vi "TcpCommunicationServerModule.vi"(7 "States":T1=enum."Status Check", 8 "エラー入力（エラーなし）":errorcluster, 10 "ポート":u16=8501) -> (0 "エラー出力":errorcluster, 1 "接続数":i32, 3 "Data出力":T2, 5 "Stoped":bool)   [LabVIEW 2017]
uses:
  TcpCommunicationServerData.ctl
  TcpCommunicationServerCMD.ctl
panel:
  out "ReadData":string
  # "サーバ用TCP通信モジュール"
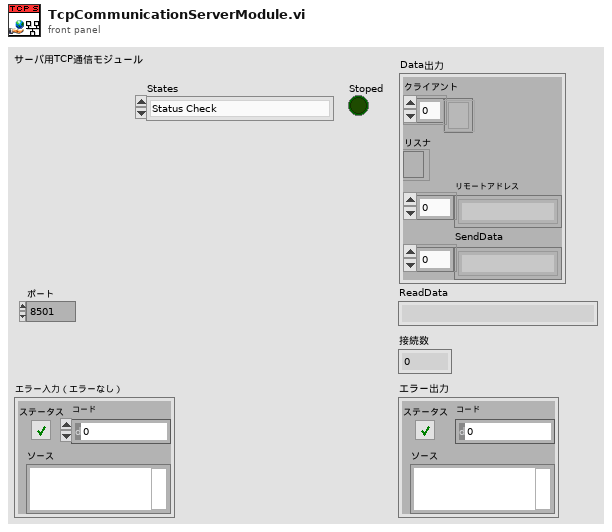
[diagram p1: front panel]
types:
  T1 = typedef "TcpCommunicationServerCMD.ctl" = enum16{"Initialize", "Status Check", "Send Data", "Read Data", "Stop", "GetData"}
  T2 = typedef "TcpCommunicationServerData.ctl" = cluster{"クライアント":refnum<k5>[], "リスナ":refnum<k5>, "リモートアドレス":string[], "SendData":string[]}
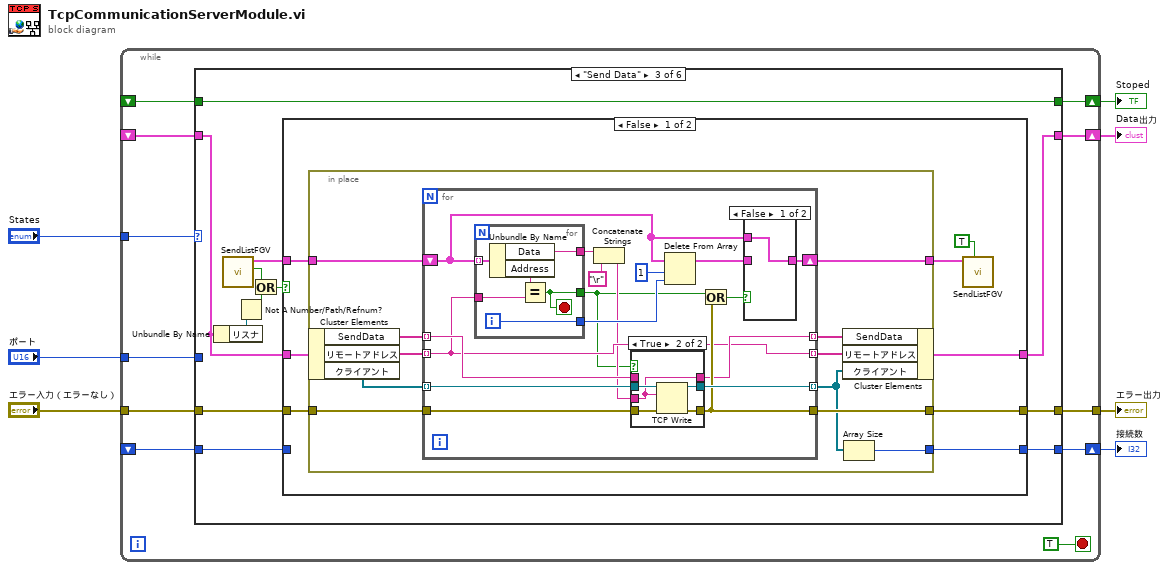
[diagram p0: block diagram]
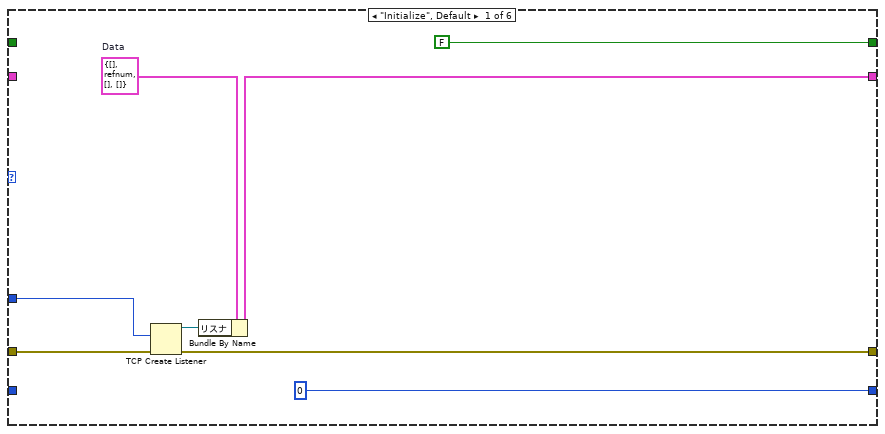
[diagram p2: hidden frame]
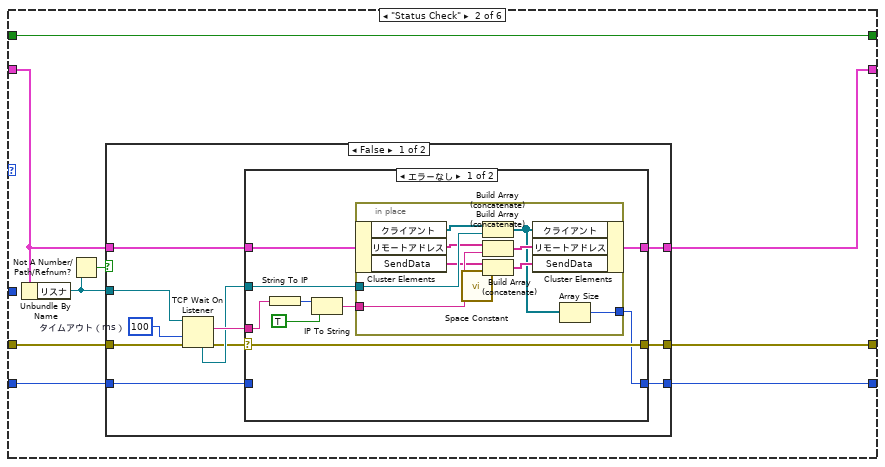
[diagram p3: hidden frame]
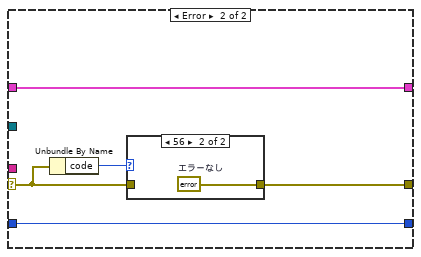
[diagram p4: hidden frame]
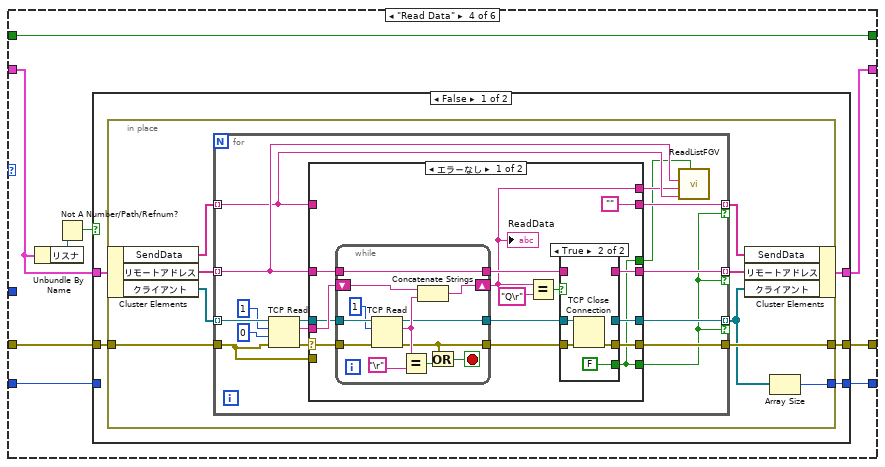
[diagram p10: hidden frame]
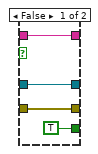
[diagram p11: hidden frame]
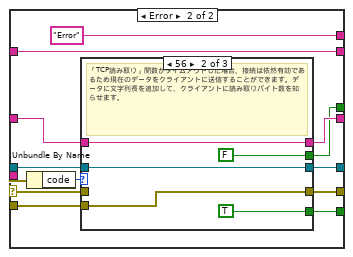
[diagram p12: hidden frame]
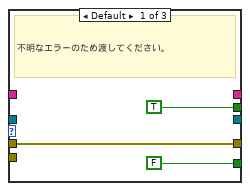
[diagram p13: hidden frame]
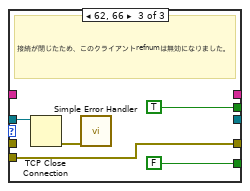
[diagram p14: hidden frame]
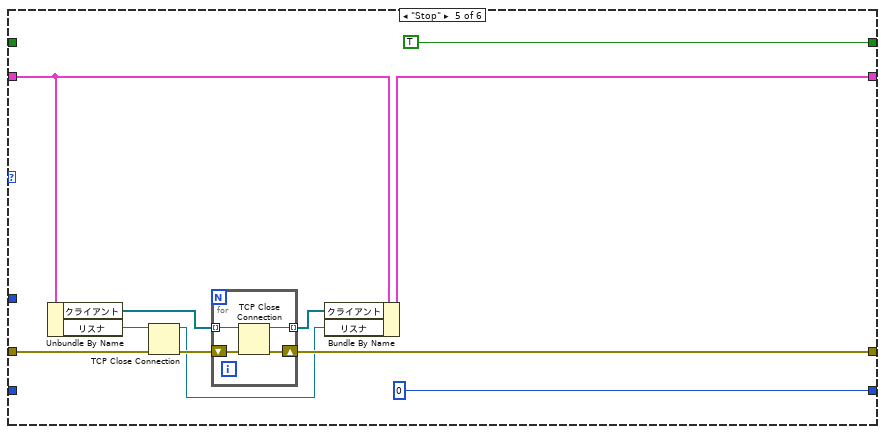
[diagram p16: hidden frame]
diagram:
  n1 = while {
    tunnel: "ポート" -> [w18]
    shift-right: [w17] -> w6
    shift-left: _ -> [w16]
    tunnel: "States" -> [w12]
    shift-right: [w10] -> w1
    shift-left: _ -> [w9]
    shift-right: [w11] -> w2
    shift-left: _ -> [w8]
    tunnel: "エラー入力（エラーなし）" -> [w14]
    tunnel: [w15] -> w5
    stop <- TRUE stop-if-true
    n2 = case shown="\"Send Data\"" w12 {
      tunnel: w18 -> [w26 _ _ _ _ _]
      tunnel: [w24 w34 w83 w148 w247 w262] -> w17
      tunnel: w16 -> [_ w32 w79 w145 w251 w262]
      tunnel: [w23 w33 w84 w150 w250 w261] -> w15
      tunnel: w14 -> [w22 w35 w85 w151 w252 w261]
      tunnel: [0 w31 w82 w149 0 w260] -> w11
      tunnel: [FALSE w30 w81 w147 TRUE w263] -> w10
      tunnel: w9 -> [_ w30 w81 w147 _ w263]
      tunnel: w8 -> [_ w29 w80 w143 _ w260]
      frame "Initialize", Default {
        w21 = T2 {"クライアント"=[], "リスナ"=refnum, "リモートアドレス"=[], "SendData"=[]}  # Data
        n3 = TCP Create Listener(8:w22, 10:w26) -> (0:w23:errorcluster, 3:w25:refnum<k5>)  [unwired: 4 out]
        n4 = Bundle By Name(cluster=w21, "リスナ"=w25) -> (w24:T2)
      }
      frame "Status Check" {
        n5 = Unbundle By Name(w32) -> ("リスナ"=w27:refnum<k5>)
        n6 = Not A Number/Path/Refnum?(number/path/refnum=w27) -> (NaN/Path/Refnum?=w28:bool)
        n7 = case shown="FALSE" w28 {
          tunnel: w27 -> [w45 _]
          tunnel: w35 -> [w41 w74]
          tunnel: [w40 w75] -> w34
          tunnel: [w39 w74] -> w33
          tunnel: w32 -> [w38 w75]
          tunnel: [w37 w73] -> w31
          tunnel: w29 -> [w36 w73]
          frame False {
            w42 = 100  # タイムアウト（ms）
            n8 = TCP Wait On Listener(8:w41, 9:w42, 11:w45) -> (0:w43:errorcluster, 2:w46:string, 4:w44:refnum<k5>)  [unwired: 3 out]
            n9 = case shown="エラーなし" w43 {
              selector: w43 -> [w53 w70]
              tunnel: w44 -> [w54 _]
              tunnel: w38 -> [w55 w67]
              tunnel: [w52 w67] -> w40
              tunnel: [w53 w68] -> w39
              tunnel: w46 -> [w49 _]
              tunnel: [w47 w66] -> w37
              tunnel: w36 -> [_ w66]
              frame No Error {
                # "新規クライアント接続をステートデータに追加して、「データを送信」ステートに進みます。"
                n10 = String To IP(1:w49) -> (0:w51:u32)
                n11 = IP To String(1:TRUE ("ドット表記法?（F）"), 2:w51) -> (0:w48:string)
                n12 = in-place {
                  in-place-border: w54 -> [w64]
                  in-place-border: w48 -> [w61]
                  in-place-border: [w56] -> w47
                  n13 = in-place-cluster #1(w55) -> ("クライアント"=w65:refnum<k5>[], "リモートアドレス"=w63:string[], "SendData"=w59:string[])
                  n14 = call <vilib>:"Space Constant.vi"() -> ("String"=w58:string)
                  n15 = Build Array (concatenate)(w65, w64) -> (w57:refnum<k5>[])
                  n16 = Build Array (concatenate)(w63, w61) -> (w62:string[])
                  n17 = Build Array (concatenate)(w59, w58) -> (w60:string[])
                  n18 = in-place-cluster #1("クライアント"=w57, "リモートアドレス"=w62, "SendData"=w60) -> (w52:T2)
                  n19 = Array Size(array=w57) -> (size(s)=w56:i32)
                }
              }
              frame Error {
                # "タイムアウトエラーを無視します。クライアントが存在する場合は、「データを送信」ステートに進みます。"
                n20 = Unbundle By Name(w70) -> ("code"=w69:i32)
                n21 = case shown="56" w69 {
                  tunnel: w70 -> [w71 _]
                  tunnel: [w71 w72] -> w68
                  frame Default {
                  }
                  frame 56 {
                    w72 = errorcluster {"status"=FALSE, "code"=0, "source"=""}  # エラーなし
                  }
                }
              }
            }
          }
          frame True {
          }
        }
      }
      frame "Send Data" {
        n22 = Unbundle By Name(w79) -> ("リスナ"=w78:refnum<k5>)
        n23 = call "SendListFGV.vi"() -> ("空?"=w86:bool, "Send List Out"=w87:cluster{"Address":string, "Data":string}[])  [unwired: 9 in, 1 out]
        n24 = Not A Number/Path/Refnum?(number/path/refnum=w78) -> (NaN/Path/Refnum?=w76:bool)
        n25 = Or(x=w86, y=w76) -> (x .or. y?=w77:bool)
        n26 = case shown="FALSE" w77 {
          tunnel: w85 -> [w95 w142]
          tunnel: [w94 w142] -> w84
          tunnel: w79 -> [w93 w141]
          tunnel: [w92 w141] -> w83
          tunnel: w87 -> [w90 _]
          tunnel: [w91 w140] -> w82
          tunnel: w80 -> [_ w140]
          frame False {
            n27 = in-place {
              in-place-border: w95 -> [w106]
              in-place-border: [w105] -> w94
              in-place-border: [w98] -> w91
              in-place-border: w90 -> [w97]
              in-place-border: [w96] -> w88
              n28 = in-place-cluster #2(w93) -> ("SendData"=w99:string[], "リモートアドレス"=w102:string[], "クライアント"=w104:refnum<k5>[])
              n29 = for {
                tunnel: w104 -> [w123] mode=indexing
                tunnel: [w122] -> w103 mode=indexing
                tunnel: w102 -> [w117] mode=indexing
                tunnel: [w117] -> w101 mode=indexing
                tunnel: [w119] -> w100 mode=indexing
                tunnel: w99 -> [w118] mode=indexing
                tunnel: w106 -> [w121]
                tunnel: [w120] -> w105
                shift-right: [w109] -> w96
                shift-left: w97 -> [w110]
                n30 = for {
                  tunnel: w110 -> [w128] mode=indexing
                  tunnel: w117 -> [w131]
                  tunnel: [w129] -> w116
                  tunnel: [w127] -> w107
                  tunnel: [w126] -> w114
                  i -> [w126]
                  stop <- w127 stop-if-true
                  n31 = Unbundle By Name(w128) -> ("Data"=w129:string, "Address"=w130:string)
                  n32 = Equal?(x=w130, y=w131) -> (x = y?=w127:bool)
                }
                n33 = Concatenate Strings(w116, "\r") -> (w112:string)
                n34 = case shown="TRUE" w107 {
                  tunnel: w123 -> [w134 w139]
                  tunnel: [w134 w138] -> w122
                  tunnel: [w133 w137] -> w120
                  tunnel: w121 -> [w133 w136]
                  tunnel: w112 -> [_ w135]
                  tunnel: w118 -> [w132 _]
                  tunnel: [w132 w135] -> w119
                  frame False {
                  }
                  frame True {
                    n35 = TCP Write(connection ID=w139, data in=w135, error in (no error)=w136) -> (connection ID out=w138:refnum<k5>, error out=w137:errorcluster)  [unwired: 2 out]
                  }
                }
                n36 = Delete From Array(array=w110, length=1 ("長さ"), index=w114) -> (array with subset deleted=w111:cluster{"Address":string, "Data":string}[])  [unwired: 1 out]
                n37 = Or(x=w107, y=w120) -> (x .or. y?=w108:bool)
                n38 = case shown="FALSE" w108 {
                  tunnel: w110 -> [w124 _]
                  tunnel: [w124 w125] -> w109
                  tunnel: w111 -> [_ w125]
                  frame False {
                  }
                  frame True {
                  }
                }
              }
              n39 = in-place-cluster #2("SendData"=w100, "リモートアドレス"=w101, "クライアント"=w103) -> (w92:T2)
              n40 = Array Size(array=w103) -> (size(s)=w98:i32)
            }
            n41 = call "SendListFGV.vi"("Set"=TRUE, "Send List"=w88) -> ()  [unwired: 7 in, 3 out]
          }
          frame True {
          }
        }
      }
      frame "Read Data" {
        n42 = Unbundle By Name(w145) -> ("リスナ"=w146:refnum<k5>)
        n43 = Not A Number/Path/Refnum?(number/path/refnum=w146) -> (NaN/Path/Refnum?=w144:bool)
        n44 = case shown="FALSE" w144 {
          tunnel: w151 -> [w156 w243]
          tunnel: [w155 w243] -> w150
          tunnel: [w154 w242] -> w149
          tunnel: w145 -> [w153 w244]
          tunnel: [w152 w244] -> w148
          tunnel: w143 -> [_ w242]
          frame False {
            n45 = in-place {
              in-place-border: w156 -> [w165]
              in-place-border: [w164] -> w155
              in-place-border: [w157] -> w154
              n46 = in-place-cluster #3(w153) -> ("SendData"=w160:string[], "リモートアドレス"=w162:string[], "クライアント"=w163:refnum<k5>[])
              n47 = for {
                tunnel: w163 -> [w181] mode=indexing
                tunnel: [w175] -> w158 mode=indexing if=w168
                tunnel: w162 -> [w172] mode=indexing
                tunnel: [w171] -> w161 mode=indexing if=w168
                tunnel: w160 -> [w170] mode=indexing
                tunnel: [w169] -> w159 mode=indexing if=w168
                tunnel: w165 -> [w173]
                tunnel: [w174] -> w164
                n48 = TCP Read(connection ID=w181, bytes to read=1 ("読み取りバイト数"), error in (no error)=w173, 9:0 ("タイムアウト")) -> (connection ID out=w180:refnum<k5>, data out=w176:string, error out=w177:errorcluster)  [unwired: 1 out]
                n49 = case shown="エラーなし" w177 {
                  selector: w177 -> [w194 w227]
                  tunnel: w180 -> [w195 w224]
                  tunnel: w176 -> [w196 _]
                  tunnel: [w192 w222] -> w175
                  tunnel: [w184 w223] -> w168
                  tunnel: [w190 w226] -> w174
                  tunnel: w173 -> [_ w225]
                  tunnel: [w188 w221] -> w171
                  tunnel: w172 -> [w185 w220]
                  tunnel: [w184 w219] -> w166
                  tunnel: w170 -> [_ w218]
                  tunnel: ["" w218] -> w169
                  tunnel: [w183 "Error"] -> w167
                  frame No Error {
                    # "クライアントがデータを送信した場合、接続を閉じる必要があることを示しています。"
                    n50 = while {
                      shift-right: [w205] -> w183
                      shift-left: w196 -> [w212]
                      tunnel: w195 -> [w216]
                      tunnel: w194 -> [w215]
                      tunnel: [w206] -> w191
                      tunnel: [w210] -> w189
                      tunnel: w185 -> [w210]
                      tunnel: [w209] -> w193
                      stop <- w207 stop-if-true
                      n51 = TCP Read(connection ID=w216, bytes to read=1 ("読み取りバイト数"), error in (no error)=w215) -> (connection ID out=w209:refnum<k5>, data out=w211:string, error out=w206:errorcluster)  [unwired: 1 in, 1 out]
                      n52 = Equal?(x=w211, y="\r") -> (x = y?=w208:bool)
                      n53 = Concatenate Strings(w212, w211) -> (w205:string)
                      n54 = Or(x=w206, y=w208) -> (x .or. y?=w207:bool)
                    }
                    "ReadData" <- w183
                    n55 = Equal?(x=w183, y="Q\r" ("x")) -> (x = y?=w187:bool)
                    n56 = case shown="TRUE" w187 {
                      tunnel: w193 -> [w198 w204]
                      tunnel: [w198 _] -> w192
                      tunnel: w191 -> [w199 w203]
                      tunnel: [w199 w202] -> w190
                      tunnel: [TRUE FALSE] -> w184
                      tunnel: w189 -> [w197 _]
                      tunnel: [w197 _] -> w188
                      frame False {
                      }
                      frame True {
                        n57 = TCP Close Connection(connection ID=w204, error in (no error)=w203) -> (error out=w202:errorcluster)  [unwired: 1 in, 1 out]
                      }
                    }
                  }
                  frame Error {
                    # "閉じられた接続とタイムアウトエラーを無視する"
                    n58 = Unbundle By Name(w227) -> ("code"=w228:i32)
                    n59 = case shown="56" w228 {
                      tunnel: w227 -> [w231 _ _]
                      tunnel: [w231 w234 w241] -> w226
                      tunnel: w225 -> [_ w234 w241]
                      tunnel: w224 -> [_ w236 w239]
                      tunnel: [FALSE TRUE FALSE] -> w223
                      tunnel: [_ w236 _] -> w222
                      tunnel: [_ w233 _] -> w221
                      tunnel: w220 -> [_ w233 _]
                      tunnel: [TRUE FALSE TRUE] -> w219
                      frame Default {
                        # "不明なエラーのため渡してください。"
                      }
                      frame 56 {
                        # "「TCP読み取り」関数がタイムアウトした場合、接続は依然有効であるため現在のデータをクライアントに送信することができます。データに文字列長を追加して、クライアントに読み取りバイト数を知らせます。"
                      }
                      frame 62, 66 {
                        # "接続が閉じたため、このクライアントrefnumは無効になりました。"
                        n60 = TCP Close Connection(connection ID=w239) -> (error out=w238:errorcluster)  [unwired: 2 in, 1 out]
                        n61 = call <vilib>:"Simple Error Handler.vi"("error in (no error)"=w238) -> ()  [unwired: 4 in, 5 out]
                      }
                    }
                  }
                }
                n62 = call "ReadListFGV.vi"("Set"=w166, "SendData"=w170, "Data"=w167, "アドレス"=w172) -> ()  [unwired: 5 in, 3 out]
              }
              n63 = in-place-cluster #3("SendData"=w159, "リモートアドレス"=w161, "クライアント"=w158) -> (w152:T2)
              n64 = Array Size(array=w158) -> (size(s)=w157:i32)
            }
          }
          frame True {
          }
        }
      }
      frame "Stop" {
        n65 = Unbundle By Name(w251) -> ("クライアント"=w253:refnum<k5>[], "リスナ"=w255:refnum<k5>)
        n66 = TCP Close Connection(connection ID=w255, error in (no error)=w252) -> (connection ID out=w246:refnum<k5>, error out=w254:errorcluster)  [unwired: 1 in]
        n67 = for {
          shift-right: [w258] -> w250
          shift-left: w254 -> [w259]
          tunnel: w253 -> [w257] mode=indexing
          tunnel: [w256] -> w245 mode=indexing
          n68 = TCP Close Connection(connection ID=w257, error in (no error)=w259) -> (connection ID out=w256:refnum<k5>, error out=w258:errorcluster)  [unwired: 1 in]
        }
        n69 = Bundle By Name(cluster=w251, "クライアント"=w245, "リスナ"=w246) -> (w247:T2)
      }
      frame "GetData" {
      }
    }
  }
  "Data出力" <- w6
  "エラー出力" <- w5
  "接続数" <- w2
  "Stoped" <- w1
